vi "DaQ_FGV.vi"(8 "Error In":errorcluster, 9 "V/A?":string, 10 "Output Signal":waveform(dbl)={"t0"=timestamp(0 s since 1904-01-01), "dt"=0.0, "Y"=[]}, 11 "Action":T1(ring)) -> (0 "Error Out":errorcluster)   [LabVIEW 2021, in "Main.lvlib"]
doc: "This FGV is used to:\n-Init DaQ process depending on the unit that is calibrated \n-Start the DaQ process\n-Stop the DaQ process\n-Delete the DaQ process \n-Remeber the Unit that is calibrated"
uses:
  Main.lvlib
  Globals/CH1.vi
  <vilib>/DAQmx/create/channels.llb/DAQmx Create Channel (AO-Current-Basic).vi
  <vilib>/DAQmx/create/channels.llb/DAQmx Create Channel (AO-Voltage-Basic).vi
  <vilib>/DAQmx/write.llb/DAQmx Write (Analog Wfm 1Chan NSamp).vi
panel:
  # "Input"
  # "Output"
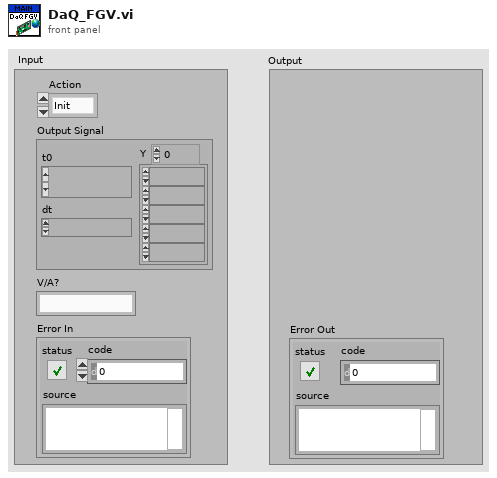
[diagram p1: front panel]
types:
  T1 = enum16{"Init", "Init DaQ", "Start", "Output", "Stop", "Delete", "V/A ?"}
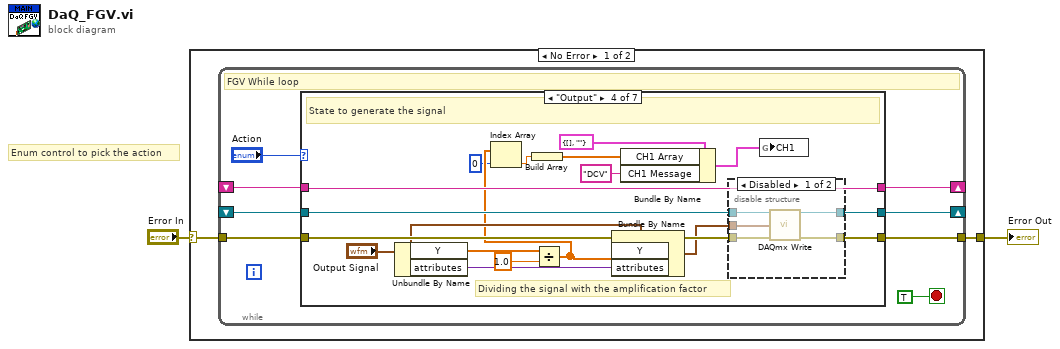
[diagram p0: block diagram]
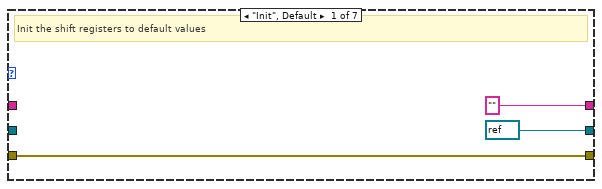
[diagram p2: hidden frame]
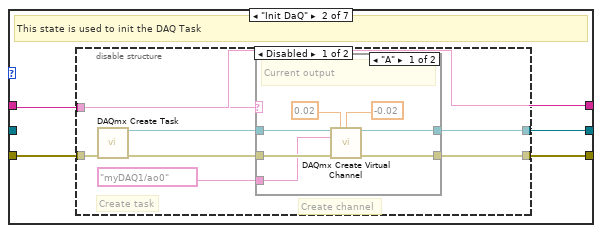
[diagram p3: hidden frame]
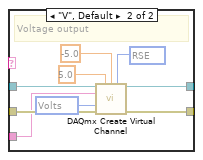
[diagram p4: hidden frame]
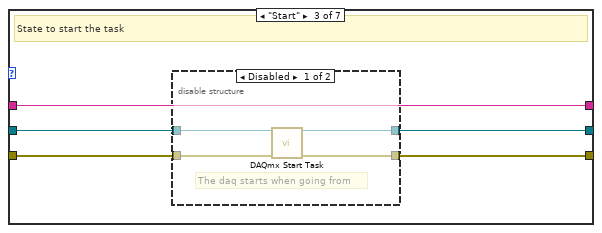
[diagram p6: hidden frame]
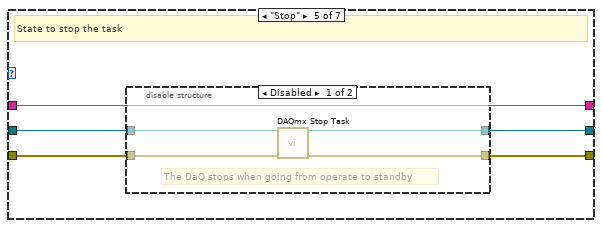
[diagram p9: hidden frame]
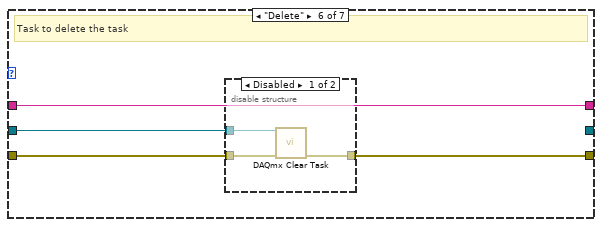
[diagram p11: hidden frame]
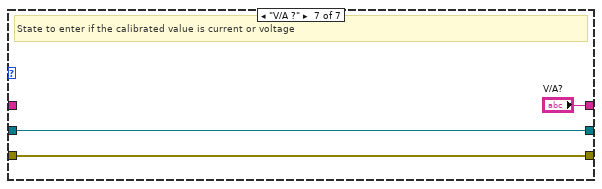
[diagram p13: hidden frame]
diagram:
  # "Enum control to pick the action"
  n1 = case shown="No Error" "Error In" {
    selector: "Error In" -> [w4 w93]
    tunnel: [w3 w93] -> w1
    frame No Error {
      n2 = while {
        shift-right: [w10] -> _
        shift-left: _ -> [w5]
        tunnel: w4 -> [w9]
        shift-right: [w8] -> _
        shift-left: _ -> [w7]
        tunnel: [w6] -> w3
        stop <- TRUE stop-if-true
        # "FGV While loop"
        n3 = case shown="\"Output\"" "Action" {
          tunnel: ["" w18 w47 w68 w78 w83 "V/A?"] -> w10
          tunnel: w9 -> [w13 w19 w45 w67 w77 w86 w92]
          tunnel: [refnum<k21> refnum ("task out") w17 w44 w65 w75 _ w91] -> w8
          tunnel: w7 -> [_ _ w46 w66 w76 w85 w91]
          tunnel: [w13 w16 w43 w64 w74 w84 w92] -> w6
          tunnel: w5 -> [_ w18 w47 w68 w78 w83 _]
          frame "Init", Default {
            # "Init the shift registers to default values"
          }
          frame "Init DaQ" {
            # "This state is used to init the DAQ Task"
            n4 = disable-structure shown="Disabled" {
              disable-tunnel: w19 -> [w26 _]
              disable-tunnel: w18 -> [w23 _]
              disable-tunnel: [w21 _] -> w17
              disable-tunnel: [w20 _] -> w16
              frame Disabled {
                # "Create channel"
                # "Create task"
                n5 = call <vilib>:"DAQmx Create Task.vi"("error in"=w26) -> ("task out"=w24:refnum<k21>, "error out"=w25:errorcluster)  [unwired: 13 in]
                n6 = case shown="\"A\"" w23 {
                  tunnel: w25 -> [w30 w42]
                  tunnel: w24 -> [w33 w41]
                  tunnel: [w32 w38] -> w21
                  tunnel: [w31 w37] -> w20
                  tunnel: tag "myDAQ1/ao0" ("physical channels") -> [w29 w36]
                  frame "A" {
                    # "Current output"
                    n7 = call-poly <vilib>:"DAQmx Create Virtual Channel.vi"("task in"=w33, "maximum value"=0.02, "minimum value"=-0.02, "physical channels"=w29, "error in"=w30) -> ("task out"=w32:refnum<k21>, "error out"=w31:errorcluster)  [unwired: 9 in]
                  }
                  frame "V", Default {
                    w39 = 10348 items=["Volts"=10348, "From Custom Scale"=10065] ("units")
                    w40 = 10083 items=["Default"=-1, "RSE"=10083, "Differential"=10106, "Pseudodifferential"=12529] ("output terminal configuration")
                    # "Voltage output"
                    n8 = call-poly <vilib>:"DAQmx Create Virtual Channel.vi"("task in"=w41, "maximum value"=5.0, "minimum value"=-5.0, "output terminal configuration"=w40, "physical channels"=w36, "units"=w39, "error in"=w42) -> ("task out"=w38:refnum<k21>, "error out"=w37:errorcluster)  [unwired: 7 in]
                  }
                }
              }
              frame Enabled {
              }
            }
          }
          frame "Start" {
            # "State to start the task"
            n9 = disable-structure shown="Disabled" {
              disable-tunnel: w46 -> [w51 _]
              disable-tunnel: w45 -> [w50 _]
              disable-tunnel: [w49 _] -> w44
              disable-tunnel: [w48 _] -> w43
              frame Disabled {
                # "The daq starts when going from"
                n10 = call <vilib>:"DAQmx Start Task.vi"("task/channels in"=w51, "error in"=w50) -> ("task out"=w49:refnum<k21>, "error out"=w48:errorcluster)  [unwired: 12 in]
              }
              frame Enabled {
              }
            }
          }
          frame "Output" {
            # "Dividing the signal with the amplification factor"
            # "State to generate the signal"
            n11 = Unbundle By Name("Output Signal") -> ("Y"=w63:dbl[], "attributes"=w61:variant)
            n12 = Divide(x=w63, y=1.0) -> (x/y=w55:dbl[])
            n13 = Index Array(array=w55, index=0) -> (element=w53:dbl)
            n14 = Build Array(w53) -> (w52:dbl[])
            n15 = Bundle By Name(cluster="Output Signal", "Y"=w55, "attributes"=w61) -> (w60:waveform(dbl))
            n16 = Bundle By Name(cluster=cluster{"CH1 Array":dbl[], "CH1 Message":string} {"CH1 Array"=[], "CH1 Message"=""} ("CH1"), "CH1 Array"=w52, "CH1 Message"="DCV") -> (w57:cluster{"CH1 Array":dbl[], "CH1 Message":string})
            n17 = disable-structure shown="Disabled" {
              disable-tunnel: w67 -> [w73 _]
              disable-tunnel: w66 -> [w72 _]
              disable-tunnel: [w71 _] -> w65
              disable-tunnel: [w70 _] -> w64
              disable-tunnel: w60 -> [w69 _]
              frame Disabled {
                n18 = call-poly <vilib>:"DAQmx Write.vi"("task/channels in"=w72, "data"=w69, "error in"=w73) -> ("task out"=w71:refnum<k21>, "error out"=w70:errorcluster)  [unwired: 10 in, 1 out]
              }
              frame Enabled {
              }
            }
            n19 = global write "CH1.vi" "CH1"(w57) -> ()
          }
          frame "Stop" {
            # "State to stop the task"
            n20 = disable-structure shown="Disabled" {
              disable-tunnel: w77 -> [w82 _]
              disable-tunnel: w76 -> [w81 _]
              disable-tunnel: [w80 _] -> w75
              disable-tunnel: [w79 _] -> w74
              frame Disabled {
                # "The DaQ stops when going from operate to standby"
                n21 = call <vilib>:"DAQmx Stop Task.vi"("task/channels in"=w81, "error in"=w82) -> ("task out"=w80:refnum<k21>, "error out"=w79:errorcluster)  [unwired: 12 in]
              }
              frame Enabled {
              }
            }
          }
          frame "Delete" {
            # "Task to delete the task"
            n22 = disable-structure shown="Disabled" {
              disable-tunnel: w86 -> [w89 _]
              disable-tunnel: w85 -> [w88 _]
              disable-tunnel: [w87 _] -> w84
              frame Disabled {
                n23 = call <vilib>:"DAQmx Clear Task.vi"("task in"=w88, "error in"=w89) -> ("error out"=w87:errorcluster)  [unwired: 13 in]
              }
              frame Enabled {
              }
            }
          }
          frame "V/A ?" {
            # "State to enter if the calibrated value is current or voltage"
          }
        }
      }
    }
    frame Error {
    }
  }
  "Error Out" <- w1
